vi "SRS865A--set-freq-and-get--V1.vi"(6 "delay-circle(msec)":i64, 8 "error in (no error)":errorcluster, 9 "freq in":dbl, 11 "VISA resource name":refnum<visa-resource-name>) -> (0 "error out":errorcluster, 1 "freq out":dbl, 2 "zi out (V)":cdb, 3 "VISA resource name out":refnum<visa-resource-name>)   [LabVIEW 2017]
uses:
  <instrlib>/Stanford Research SR865/Stanford Research SR865.lvlib
panel:
  out "concatenated string":string
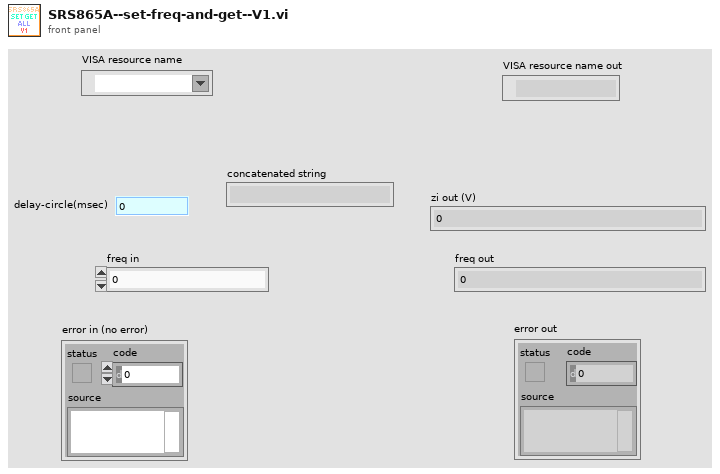
[diagram p1: front panel]
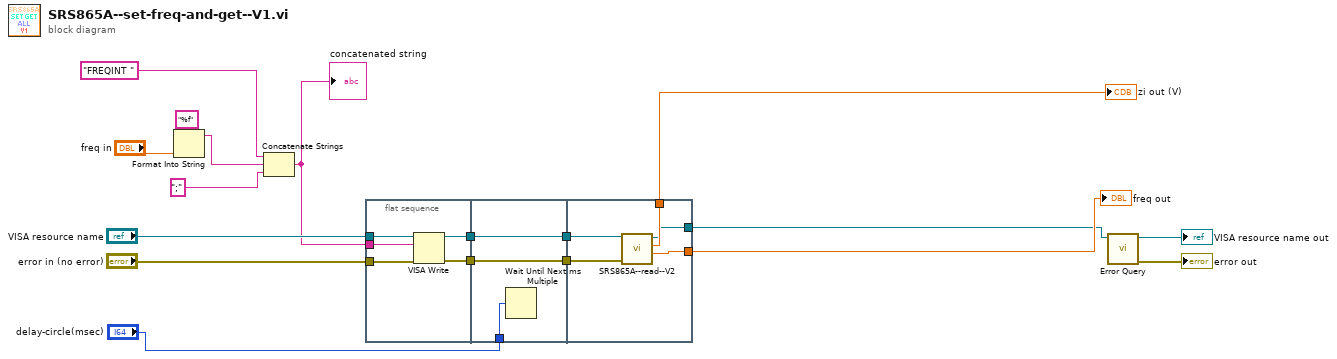
[diagram p0: block diagram]
diagram:
  n1 = Format Into String(format string="%f", "freq in") -> (resulting string=w12:string)  [unwired: 2 in, 1 out]
  n2 = Concatenate Strings("FREQINT ", w12, ";" ("format string")) -> (w10:string)
  "concatenated string" <- w10
  n3 = flat-sequence {
    tunnel: "VISA resource name" -> [w23]
    tunnel: "error in (no error)" -> [w22]
    tunnel: w10 -> [w21]
    tunnel: [w20] -> w5
    tunnel: [w19] -> w3
    tunnel: w5 -> [w26]
    tunnel: [w26] -> w4
    tunnel: w3 -> [w25]
    tunnel: [w25] -> w2
    tunnel: "delay-circle(msec)" -> [w24]
    tunnel: w4 -> [w30]
    tunnel: w2 -> [w31]
    tunnel: [w29] -> w8
    tunnel: [w28] -> w7
    tunnel: [w27] -> w6
    frame #0 {
      n4 = VISA Write(VISA resource name=w23, write buffer=w21, error in (no error)=w22) -> (VISA resource name out=w20:refnum<visa-resource-name>, error out=w19:errorcluster)  [unwired: 1 out]
    }
    frame #1 {
      n5 = Wait Until Next ms Multiple(millisecond multiple=w24) -> ()  [unwired: 1 out]
    }
    frame #2 {
      n6 = call "SRS865A--read--V2.vi"("error in (no error)"=w31, "VISA resource name"=w30) -> ("freq out"=w29:dbl, "zi out (V)"=w28:cdb, "VISA resource name out"=w27:refnum<visa-resource-name>)  [unwired: 6 in, 1 out]
    }
  }
  n7 = call <instrlib>:"Error Query.vi"("VISA resource name"=w6) -> ("error out"=→"error out":errorcluster, "VISA resource name out"=→"VISA resource name out":refnum<visa-resource-name>)  [unwired: 8 in, 1 out]
  "freq out" <- w8
  "zi out (V)" <- w7
